vi "LUnit Start Test.vi"(8 "error in (no error)":errorcluster, 10 "Tests":string[](array[string]), 11 "Coverage Report In":refnum<class "Coverage Report.lvclass">) -> (0 "error out":errorcluster, 3 "Coverage Report Out":refnum<class "Coverage Report.lvclass">)   [LabVIEW 2020, in "Coverage Report.lvclass"]
uses:
  Coverage Report.lvclass
  Coverage Report.lvclass/Coverage Report.ctl
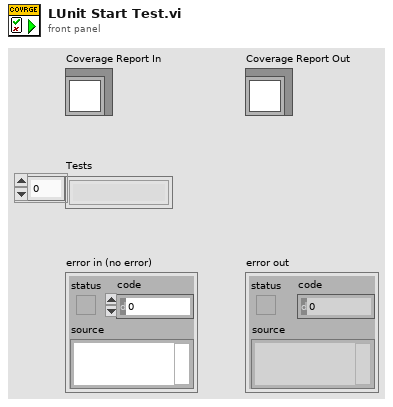
[diagram p1: front panel]
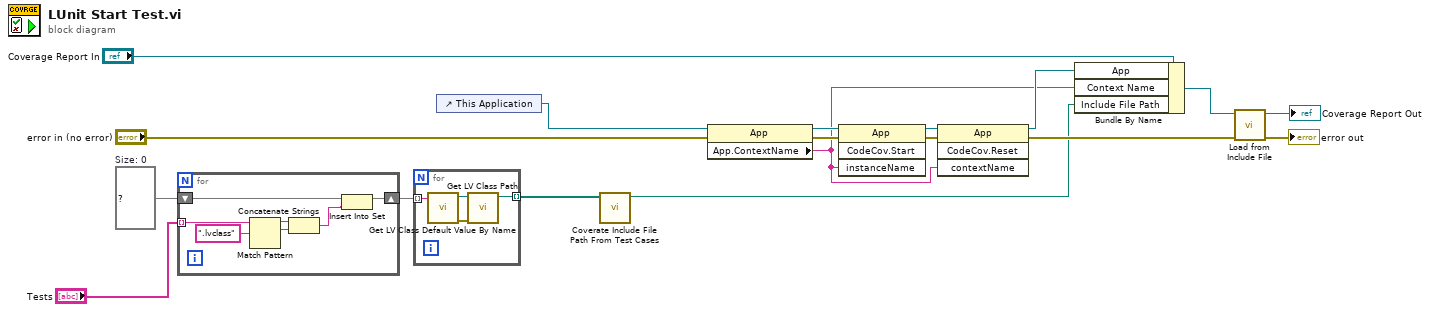
[diagram p0: block diagram]
diagram:
  w4 = set{string} {}  # Size: 0
  n1 = for {
    tunnel: "Tests" -> [w25] mode=indexing
    shift-right: [w20] -> w3
    shift-left: w4 -> [w21]
    n2 = Match Pattern(string=w25, regular expression=".lvclass") -> (before substring=w23:string, match substring=w22:string)  [unwired: 1 in, 2 out]
    n3 = Concatenate Strings(w23, w22) -> (w19:string)
    n4 = Insert Into Set(10:w19, 11:w21) -> (3:w20:set{string})  [unwired: 1 out]
  }
  n5 = for {
    tunnel: w3 -> [w29] mode=indexing
    tunnel: [w26] -> w2 mode=indexing
    n6 = call <vilib>:"Get LV Class Default Value By Name.vi"("class name"=w29) -> ("error out"=w27:errorcluster, "object"=w28:refnum<class>)  [unwired: 9 in]
    n7 = call <vilib>:"Get LV Class Path.vi"("error in (no error)"=w27, "object"=w28) -> ("class path"=w26:path)  [unwired: 8 in, 1 out]
  }
  n8 = control-ref of="This Application"() -> (w14:refnum<vi>)
  n9 = call "Coverate Include File Path From Test Cases.vi"("Test Case Classes"=w2) -> ("appended path"=w1:path)  [unwired: 10 in]
  n10 = property class="App"(reference=w14, error in="error in (no error)") -> (reference out=w11:refnum<vi>, error out=w12:errorcluster, "App.ContextName"=w10:string)
  n11 = invoke class="App" method="CodeCov.Start"(reference=w11, error in=w12, "instanceName"=w10) -> (reference out=w16:refnum<vi>, error out=w15:errorcluster)  [unwired: 1 in, 2 out]
  n12 = invoke class="App" method="CodeCov.Reset"(reference=w16, error in=w15, "contextName"=w10) -> (reference out=w17:refnum<vi>, error out=w9:errorcluster)  [unwired: 1 in, 2 out]
  n13 = Bundle By Name(cluster="Coverage Report In", "App"=w17, "Context Name"=w10, "Include File Path"=w1) -> (w7:refnum<class "Coverage Report.lvclass">)
  n14 = call "Load from Include File.vi"("error in (no error)"=w9, "Coverage Report in"=w7) -> ("error out"=→"error out":errorcluster, "Coverage Report out"=→"Coverage Report Out":refnum<class "Coverage Report.lvclass">)  [unwired: 8 in]
